vi "Construct Dual DMD Intensity Coefficients (SubVI).vi"(8 "Number of Rows Processed":refnum<vi>, 11 "Image Size in":T1={"Height"=3072, "Width"=3200}) -> ()   [LabVIEW 2017]
uses:
  Controls (HOST)/Image Size.ctl
  <vilib>/Utility/file.llb/Read Delimited Spreadsheet (DBL).vi
  <vilib>/Utility/file.llb/Write Delimited Spreadsheet (DBL).vi
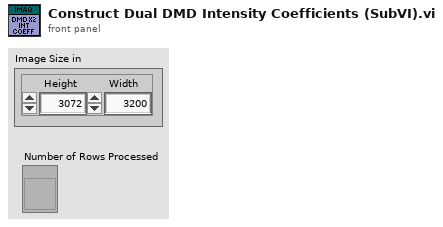
[diagram p1: front panel]
types:
  T1 = typedef "Image Size.ctl" = cluster{"Height":u16, "Width":u16}
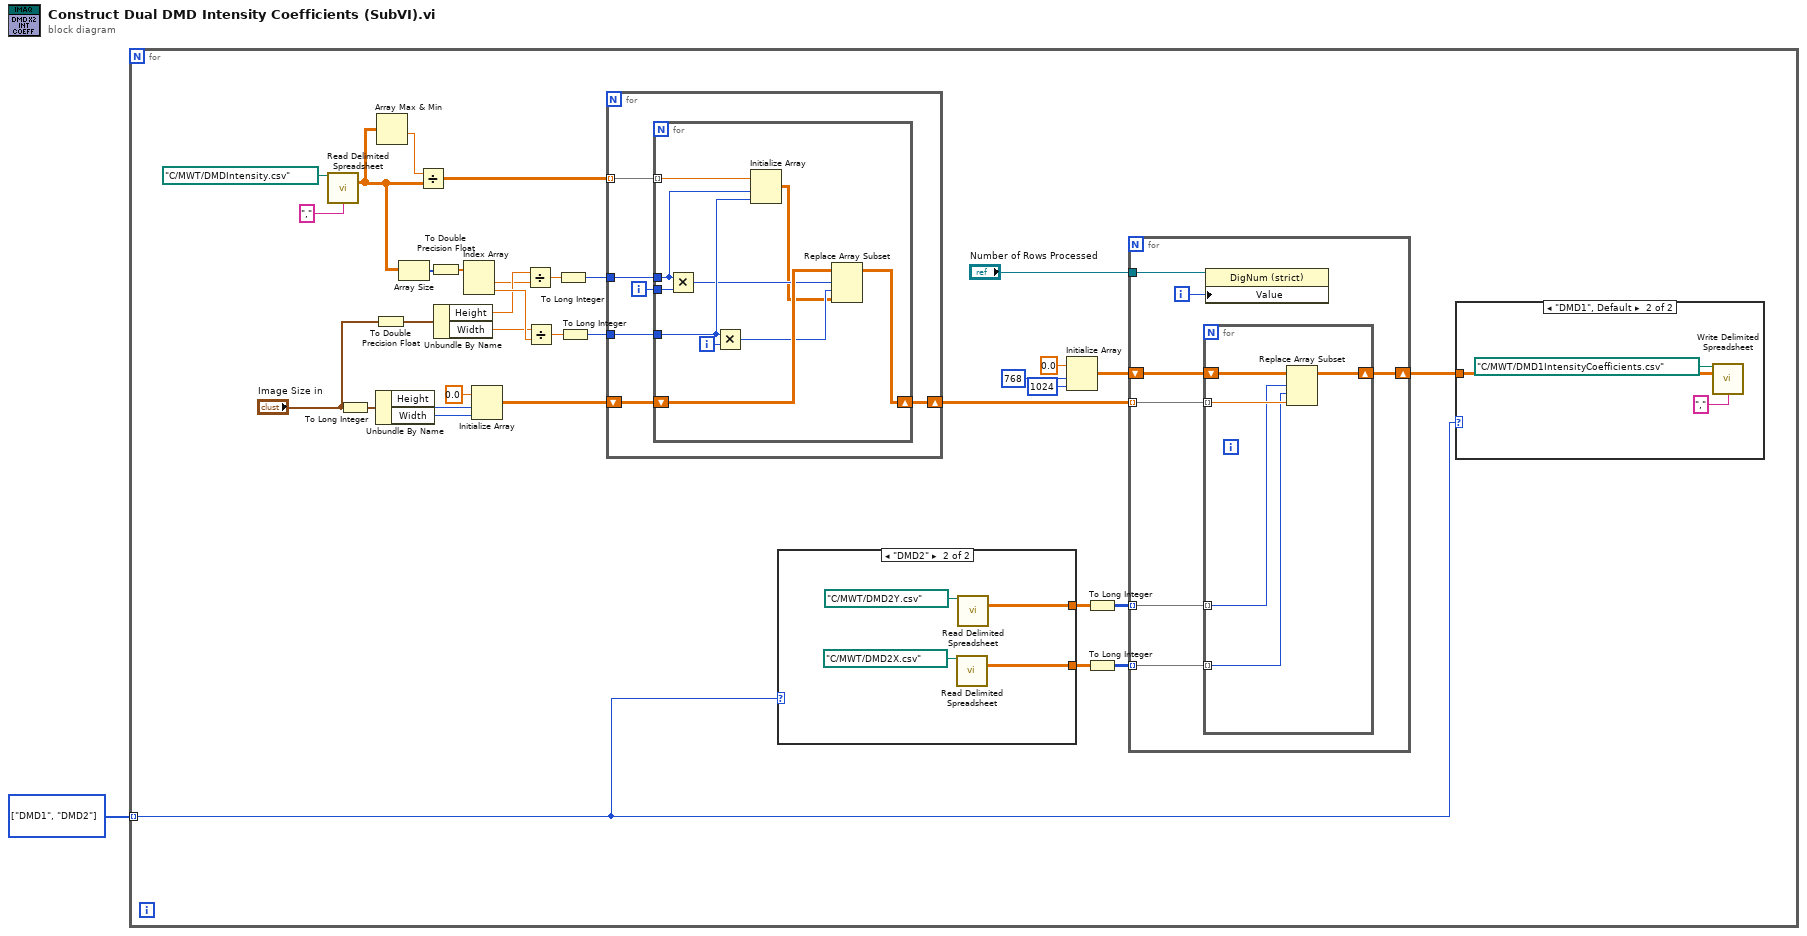
[diagram p0: block diagram]
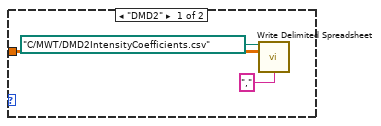
[diagram p2: hidden frame]
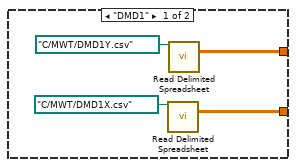
[diagram p3: hidden frame]
diagram:
  w1 = enum16{"DMD1", "DMD2"}[] [enum."DMD1", enum."DMD2"] items=["DMD1", "DMD2"]
  n1 = for {
    tunnel: w1 -> [w6] mode=indexing
    n2 = call-poly <vilib>:"Read Delimited Spreadsheet.vi"("file path (dialog if empty)"=path "C:/MWT/DMDIntensity.csv", "delimiter (\\t)"="," ("delimiter (\\t)")) -> ("all rows"=w15:dbl[][])  [unwired: 8 in, 5 out]
    n3 = To Long Integer(number="Image Size in") -> (32bit integer=w14:cluster{"Height":i32, "Width":i32})
    n4 = To Double Precision Float(number="Image Size in") -> (double precision float=w20:cluster{"Height":dbl, "Width":dbl})
    n5 = Unbundle By Name(w14) -> ("Height"=w11:i32, "Width"=w12:i32)
    n6 = Array Max & Min(array=w15) -> (min value=w10:dbl)  [unwired: 3 out]
    n7 = Array Size(array=w15) -> (size(s)=w16:i32[])
    n8 = Divide(x=w10, y=w15) -> (x/y=w18:dbl[][])
    n9 = To Double Precision Float(number=w16) -> (double precision float=w19:dbl[])
    n10 = Unbundle By Name(w20) -> ("Height"=w22:dbl, "Width"=w23:dbl)
    n11 = Index Array(array=w19) -> (element #1=w21:dbl, element #2=w24:dbl)  [unwired: 2 in]
    n12 = Initialize Array(0.0 ("element"), w11, w12) -> (w17:dbl[][])
    n13 = Divide(x=w22, y=w21) -> (x/y=w25:dbl)
    n14 = Divide(x=w23, y=w24) -> (x/y=w26:dbl)
    n15 = To Long Integer(number=w25) -> (32bit integer=w27:i32)
    n16 = To Long Integer(number=w26) -> (32bit integer=w28:i32)
    n17 = for {
      shift-right: [w65] -> w29
      shift-left: w17 -> [w66]
      tunnel: w18 -> [w67] mode=indexing
      tunnel: w27 -> [w64]
      tunnel: w28 -> [w62]
      i -> [w63]
      n18 = for {
        tunnel: w67 -> [w73] mode=indexing
        shift-right: [w74] -> w65
        shift-left: w66 -> [w75]
        tunnel: w64 -> [w72]
        tunnel: w63 -> [w77]
        tunnel: w62 -> [w71]
        i -> [w76]
        n19 = Multiply(x=w72, y=w77) -> (x*y=w70:i32)
        n20 = Multiply(x=w71, y=w76) -> (x*y=w69:i32)
        n21 = Initialize Array(w73, w72, w71) -> (w68:dbl[][])
        n22 = Replace Array Subset(array=w75, new element=w68, index (row)=w70, index (col)=w69) -> (w74:dbl[][])
      }
    }
    n23 = case shown="\"DMD2\"" w6 {
      tunnel: [w43 w47] -> w5
      tunnel: [w42 w46] -> w4
      frame "DMD1" {
        n24 = call-poly <vilib>:"Read Delimited Spreadsheet.vi"("file path (dialog if empty)"=path "C:/MWT/DMD1X.csv") -> ("all rows"=w42:dbl[][])  [unwired: 9 in, 5 out]
        n25 = call-poly <vilib>:"Read Delimited Spreadsheet.vi"("file path (dialog if empty)"=path "C:/MWT/DMD1Y.csv") -> ("all rows"=w43:dbl[][])  [unwired: 9 in, 5 out]
      }
      frame "DMD2" {
        n26 = call-poly <vilib>:"Read Delimited Spreadsheet.vi"("file path (dialog if empty)"=path "C:/MWT/DMD2X.csv") -> ("all rows"=w46:dbl[][])  [unwired: 9 in, 5 out]
        n27 = call-poly <vilib>:"Read Delimited Spreadsheet.vi"("file path (dialog if empty)"=path "C:/MWT/DMD2Y.csv") -> ("all rows"=w47:dbl[][])  [unwired: 9 in, 5 out]
      }
    }
    n28 = Initialize Array(0.0 ("element"), 768 ("dimension size"), 1024 ("dimension size")) -> (w33:dbl[][])
    n29 = To Long Integer(number=w5) -> (32bit integer=w3:i32[][])
    n30 = To Long Integer(number=w4) -> (32bit integer=w2:i32[][])
    n31 = for {
      tunnel: "Number of Rows Processed" -> [w54]
      tunnel: w29 -> [w55] mode=indexing
      shift-right: [w52] -> w7
      shift-left: w33 -> [w56]
      tunnel: w3 -> [w51] mode=indexing
      tunnel: w2 -> [w50] mode=indexing
      i -> [w53]
      n32 = for {
        tunnel: w55 -> [w59] mode=indexing
        shift-right: [w60] -> w52
        shift-left: w56 -> [w61]
        tunnel: w51 -> [w58] mode=indexing
        tunnel: w50 -> [w57] mode=indexing
        n33 = Replace Array Subset(array=w61, new element=w59, index (row)=w58, index (col)=w57) -> (w60:dbl[][])
      }
      n34 = property class="DigNum (strict)"(reference=w54, "Value"=w53) -> ()  [unwired: 1 in, 2 out]
    }
    n35 = case shown="\"DMD1\", Default" w6 {
      tunnel: w7 -> [w36 w39]
      frame "DMD2" {
        n36 = call-poly <vilib>:"Write Delimited Spreadsheet.vi"("file path (dialog if empty)"=path "C:/MWT/DMD2IntensityCoefficients.csv", "2D data"=w36, "delimiter (\\t)"="," ("delimiter (\\t)")) -> ()  [unwired: 11 in, 2 out]
      }
      frame "DMD1", Default {
        n37 = call-poly <vilib>:"Write Delimited Spreadsheet.vi"("file path (dialog if empty)"=path "C:/MWT/DMD1IntensityCoefficients.csv", "2D data"=w39, "delimiter (\\t)"="," ("delimiter (\\t)")) -> ()  [unwired: 11 in, 2 out]
      }
    }
  }
